vi "Generate Maze.vi"(8 "error in (no error)":errorcluster, 9 "Height":i32, 10 "Width":i32, 11 "Intermediate Maze in":refnum<class "Intermediate.lvclass">) -> (0 "error out":errorcluster, 2 "Maze":refnum<class "Maze.lvclass">, 3 "Intermediate Maze out":refnum<class "Intermediate.lvclass">)   [LabVIEW 2020, in "Intermediate Maze.lvlib" / "Intermediate.lvclass"]
uses:
  Intermediate.lvclass
  build/ppl/maze.lvlibp/Maze/Maze.lvclass
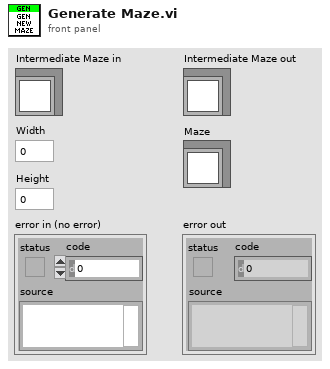
[diagram p1: front panel]
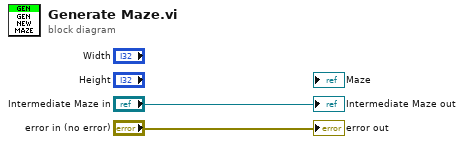
[diagram p0: block diagram]
diagram:
  "error out" <- "error in (no error)"
  "Intermediate Maze out" <- "Intermediate Maze in"
